vi "ShooterSim_Example.vi"() -> ()   [LabVIEW 2019]
uses:
  <vilib>/Rock Robotics/WPI/ThirdParty/JAS_Junk/TrajLib/DCMOTOR.CTL
  <vilib>/Rock Robotics/WPI/ThirdParty/JAS_Junk/TrajLib/LINEAR_SYSTEM.ctl
  <vilib>/Analysis/Matrix/Datatypes/RealMatrix.ctl
  <vilib>/Rock Robotics/WPI/ThirdParty/JAS_Junk/TrajLib/LINEAR_QUADRATIC_REGULATOR.ctl
  <vilib>/Rock Robotics/WPI/ThirdParty/JAS_Junk/TrajLib/KALMAN_FILTER.ctl
  <vilib>/Rock Robotics/WPI/ThirdParty/JAS_Junk/TrajLib/LINEAR_SYSTEM_LOOP.ctl
  <vilib>/Rock Robotics/WPI/ThirdParty/JAS_Junk/TrajLib/LINEAR_PLANT_INV_FF.ctl
  <vilib>/Rock Robotics/WPI/ThirdParty/JAS_Junk/TrajLib/FLYWHEEL_SIM.ctl
  <vilib>/Rock Robotics/WPI/ThirdParty/JAS_Junk/TrajLib/LINEAR_SYSTEM_SIM.ctl
  <vilib>/Rock Robotics/WPI/ThirdParty/JAS_Junk/TrajLib/DCMotor_New.vi
  <vilib>/Rock Robotics/WPI/ThirdParty/JAS_Junk/TrajLib/MatBuilder_Create.vi
  <vilib>/Rock Robotics/WPI/ThirdParty/JAS_Junk/TrajLib/LinearSystem_New.vi
  <vilib>/Rock Robotics/WPI/ThirdParty/JAS_Junk/TrajLib/MatrixHelper_Zero.vi
  <vilib>/Rock Robotics/WPI/ThirdParty/JAS_Junk/TrajLib/MatBuilder_Fill.vi
  <vilib>/Rock Robotics/WPI/ThirdParty/JAS_Junk/TrajLib/Matrix_Ident.vi
  <vilib>/Rock Robotics/WPI/ThirdParty/JAS_Junk/TrajLib/MatrixHelper_CoerceSize.vi
  <vilib>/Analysis/7linalg.llb/Create Special Matrix.vi
  <vilib>/Analysis/7linalg.llb/Create Special Real Matrix.vi
  <vilib>/Rock Robotics/WPI/ThirdParty/JAS_Junk/TrajLib/Trajectory_Library.lvlib
  <vilib>/Analysis/Matrix/NI_Matrix.lvlib
panel:
  in  "Tab Control":T1(tab)
  out "Motor Current":dbl format="%20.3f"
  out "Battery Voltage":dbl format="%20.3f"
  in  "Shoot ball":bool
  out "CO Chart":cluster{dbl, "Voltage":dbl}(graph)
  in  "Shooter On/Off":bool
  out "Encoer Speed\nRad/Sec":dbl(slide) scale=0.0..300.0
  out "Speed":dbl format="%20.3f"
  out "Cor Err":bool
  out "Kalman Filtered\nSpeed":dbl format="%20.3f"
  out "PV Chart":T2(graph)
  out "Predict Err":bool
  out "Motor Volt Dmd (CO)":dbl format="%20.3f"
  out "shoot Start":bool
  out "Shoot Done":bool
  out "Shooter Motor":T3 {"Jr_KgM2" format="%13.5p"; "L_H" format="%13.5p"; "Kt_NMPerAmp" format="%13.5p"; "KvINV_RadPerSecPerVolt" format="%13.5p"; "R_Ohms" format="%13.5p"; "FreeSpeed_RadPerSec" format="%13.5p"; "FreeCurrent_Amps" format="%13.5p"; "StallCurrent_Amps" format="%13.5p"; "StallTorque_NM" format="%13.5p"; "nominalVoltage_Volts" format="%13.5p"}
  out "m_flywheelPlant_ALT":T4
  out "m_FlyWheelSim":T6 {"GearBox"."Jr_KgM2" format="%13.5p"; "GearBox"."L_H" format="%13.5p"; "GearBox"."Kt_NMPerAmp" format="%13.5p"; "GearBox"."KvINV_RadPerSecPerVolt" format="%13.5p"; "GearBox"."R_Ohms" format="%13.5p"; "GearBox"."FreeSpeed_RadPerSec" format="%13.5p"; "GearBox"."FreeCurrent_Amps" format="%13.5p"; "GearBox"."StallCurrent_Amps" format="%13.5p"; "GearBox"."StallTorque_NM" format="%13.5p"; "GearBox"."nominalVoltage_Volts" format="%13.5p"}
  out "Shooting A":T5
  out "Shooting B":T5
  out "KalmanFilter":T8
  out "Kalman Error":errorcluster
  out "LinearQuadraticRegulator":T9
  out "LQR Error":bool
  out "Linear System Loop":T10
  out "LinSysLoop_Error":bool
  # "<States,States>"
  # "<States,Inputs>"
  # "<Outputs,States>"
  # "<Outputs,Inputs>"
  # "<States, 1>"
  # "<Outputs, 1>"
  # "<Inputs, 1>"
  # "<Outputs, 1>"
  # "<States,States>"
  # "<States,Inputs>"
  # "<Outputs,States>"
  # "<Outputs,Inputs>"
  # "Steady State Gain  \n<States,Outputs>"
  # "State Estimate <Statess,1>"
  # "<States,States>"
  # "<States,Inputs>"
  # "<Outputs,States>"
  # "<Outputs,Inputs>"
  # "Ref State <States,1>"
  # "Comp and capped \noutput <Inputs,1>"
  # "Controller gain\n<Inputs,States>"
  # "<States,1>"
  # "<FUTURE --- CLAMP TYPE -- For now\nuse Normalize>"
  # "Steady State Gain  \n<States,Outputs>"
  # "State Estimate <Statess,1>"
  # "<States,States>"
  # "<States,Inputs>"
  # "<Outputs,States>"
  # "<Outputs,Inputs>"
  # "<States,1>"
  # "<Inputs,1>"
  # "<States,Inputs>"
  # "<States,States>"
  # "Ref State <States,1>"
  # "Comp and capped \noutput <Inputs,1>"
  # "Controller gain\n<Inputs,States>"
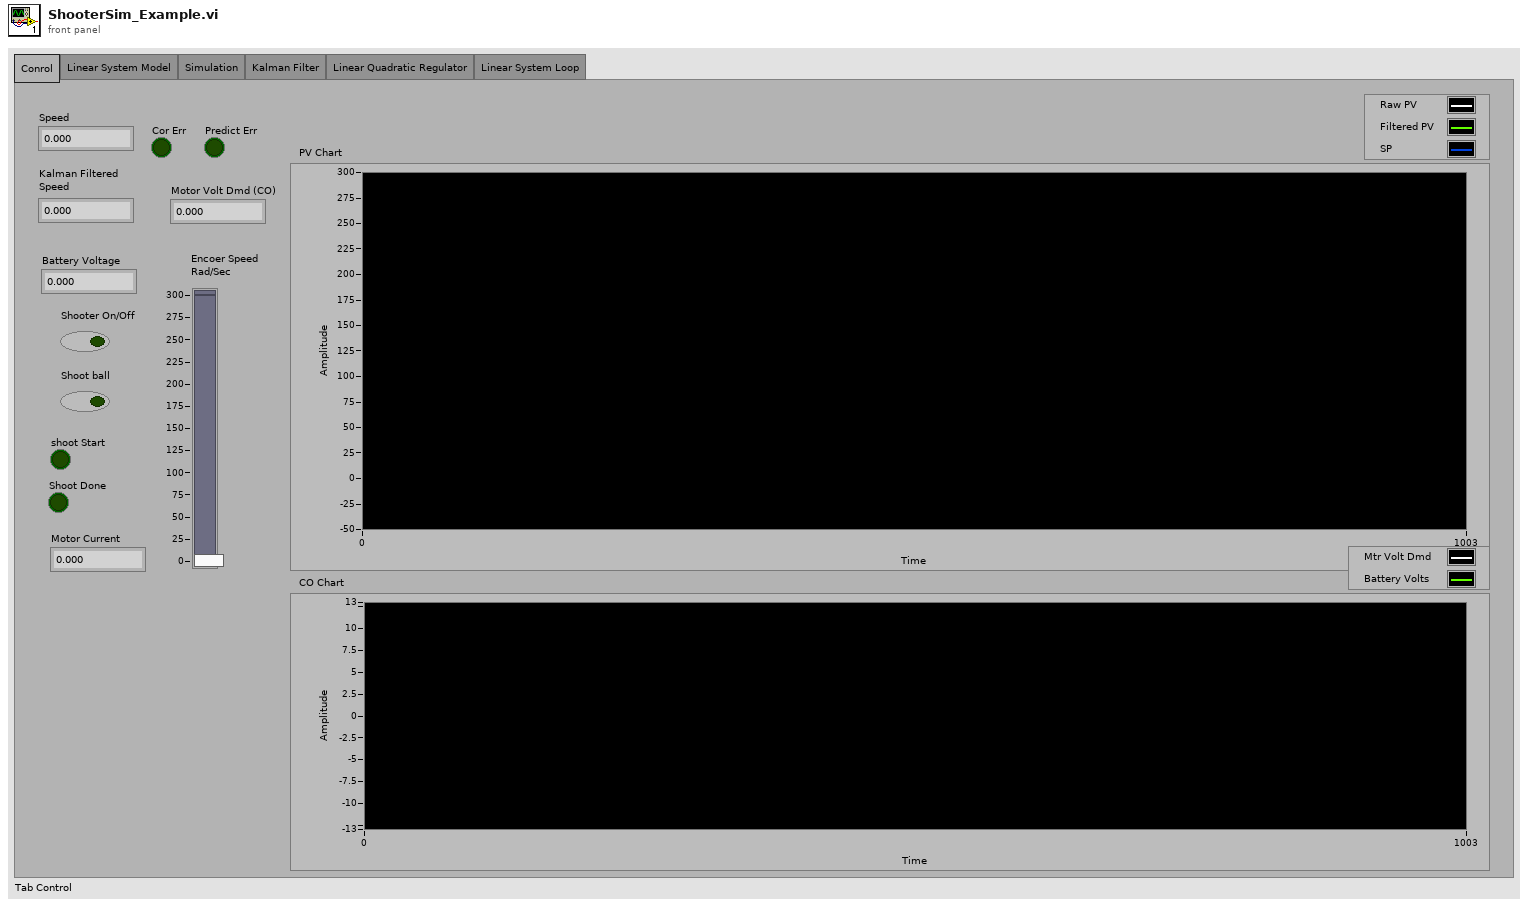
[diagram p1: front panel]
types:
  T1 = enum32{"Conrol", "Linear System Model", "Simulation", "Kalman Filter", "Linear Quadratic Regulator", "Linear System Loop"}
  T2 = cluster{"upper limit":dbl, "Real Matrix Element":dbl, "Real Matrix Element":dbl}
  T3 = typedef "Trajectory_Library.lvlib/DCMOTOR.CTL" = cluster{"nominalVoltage_Volts":dbl, "StallTorque_NM":dbl, "StallCurrent_Amps":dbl, "FreeCurrent_Amps":dbl, "FreeSpeed_RadPerSec":dbl, "R_Ohms":dbl, "KvINV_RadPerSecPerVolt":dbl, "Kt_NMPerAmp":dbl, "L_H":dbl, "Jr_KgM2":dbl}
  T4 = typedef "Trajectory_Library.lvlib/LINEAR_SYSTEM.ctl" = cluster{"m_A":T5, "m_B":T5, "m_C":T5, "m_D":T5, "States":i32, "Inputs":i32, "Outputs":i32}
  T5 = typedef "NI_Matrix.lvlib/RealMatrix.ctl" = dbl[][]
  T6 = typedef "Trajectory_Library.lvlib/FLYWHEEL_SIM.ctl" = cluster{"LinearSystemSim":T7, "GearBox":T3, "Gearing":dbl}
  T7 = typedef "Trajectory_Library.lvlib/LINEAR_SYSTEM_SIM.ctl" = cluster{"m_Plant":T4, "m_X":T5, "m_Y":T5, "m_U":T5, "MeasureStdDev":T5}
  T8 = typedef "Trajectory_Library.lvlib/KALMAN_FILTER.ctl" = cluster{"m_K":T5, "m_xHat":T5, "States":i32, "Outputs":i32, "m_Plant":T4}
  T9 = typedef "Trajectory_Library.lvlib/LINEAR_QUADRATIC_REGULATOR.ctl" = cluster{"m_r":T5, "m_U":T5, "m_K":T5, "States":i32, "Inputs":i32}
  T10 = typedef "Trajectory_Library.lvlib/LINEAR_SYSTEM_LOOP.ctl" = cluster{"Controller":T9, "FeedForward":T11, "Observer":T8, "Next_R":T5, "Clamp Max":T5}
  T11 = typedef "Trajectory_Library.lvlib/LINEAR_PLANT_INV_FF.ctl" = cluster{"m_R":T5, "m_Uff":T5, "m_B":T5, "m_A":T5, "States":i32, "Inputs":i32}
  T12 = cluster{"Velocity_RadPerSec":dbl, "Real Matrix Element":dbl, "Real Matrix Element":dbl}
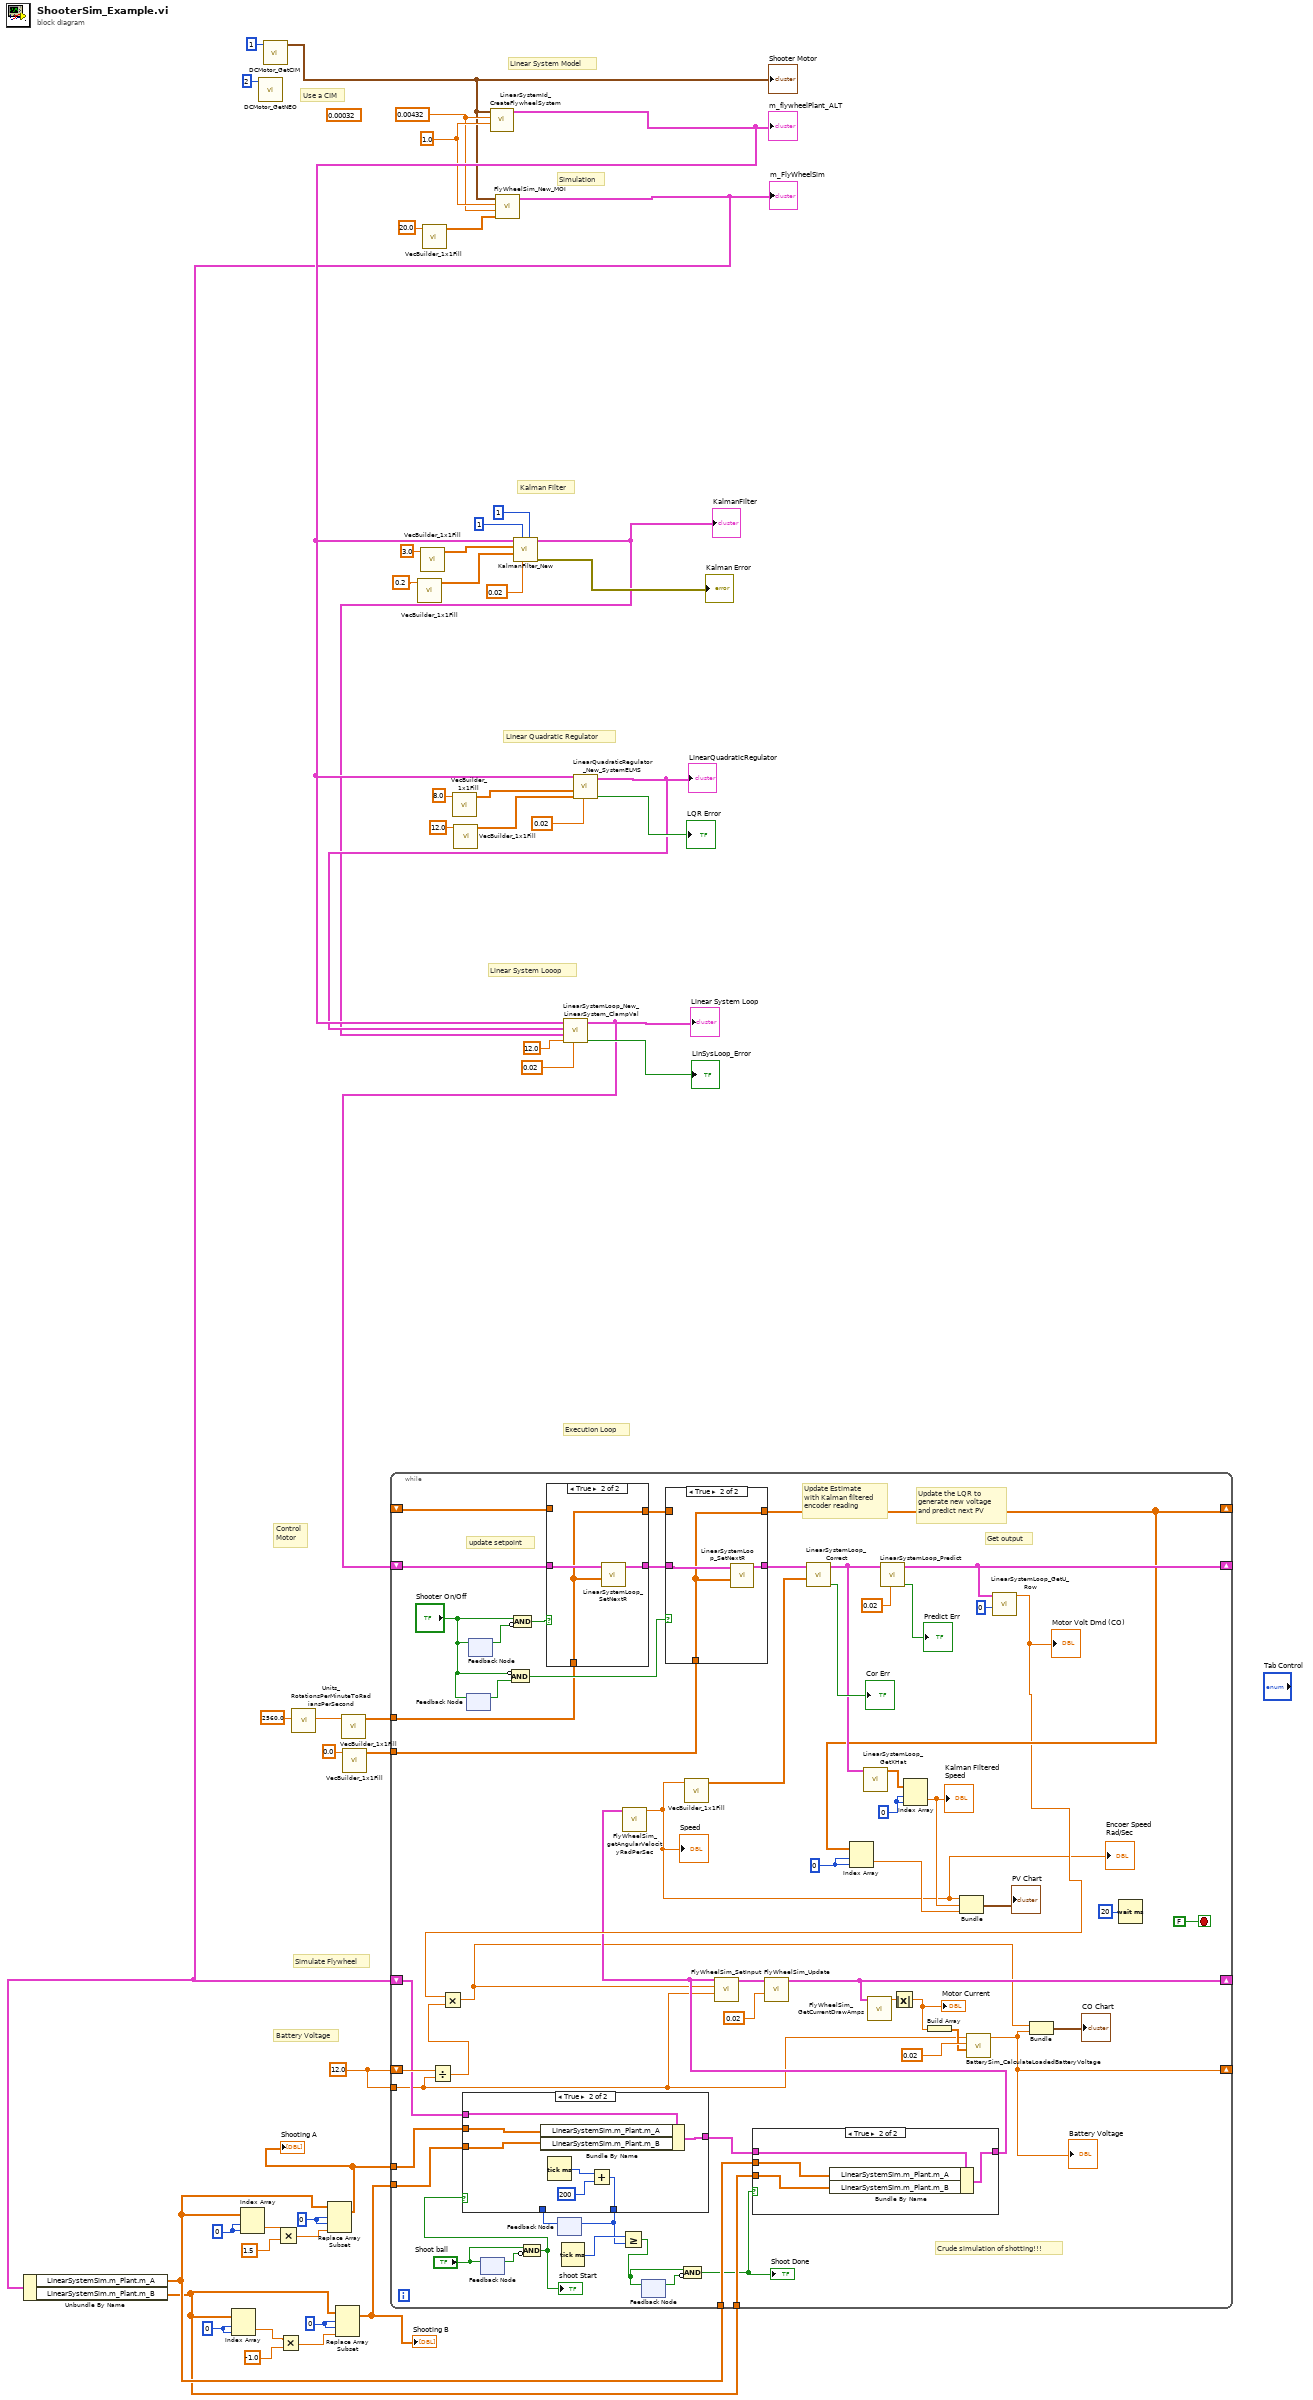
[diagram p0: block diagram]
diagram:
  w11 = 0 ("index (row)")
  w12 = 0 ("index (row)")
  w13 = 0 ("index (row)")
  w14 = 0 ("index (row)")
  w18 = 12.0
  w19 = 0.00432 ("jKgMetersSquared")
  w22 = 1.0 ("G")
  (unwired) 0.00032 ("jKgMetersSquared")
  # "Execution Loop"
  # "Linear System Looop"
  # "Linear Quadratic Regulator"
  # "Kalman Filter"
  # "Simulation"
  # "Linear System Model"
  # "Control\nMotor"
  # "Simulate Flywheel"
  # "Use a CIM"
  # "Battery Voltage"
  n1 = call <vilib>:"DCMotor_GetNEO.vi"("Num Motors"=2) -> ()  [unwired: 10 in, 1 out]
  n2 = call <vilib>:"DCMotor_GetCIM.vi"("Num Motors"=1) -> ("DCMOTOR"=w17:T3)  [unwired: 10 in]
  "Shooter Motor" <- w17
  n3 = call <vilib>:"Units_RotationsPerMinuteToRadiansPerSecond.vi"("RotationsPerMinute"=2560.0) -> ("RadiansPerSecond"=w26:dbl)  [unwired: 10 in]
  n4 = call <vilib>:"VecBuilder_1x1Fill.vi"("R0_C0"=w26) -> ("output matrix"=w24:T5)  [unwired: 10 in]
  n5 = call <vilib>:"VecBuilder_1x1Fill.vi"("R0_C0"=0.0) -> ("output matrix"=w23:T5)  [unwired: 10 in]
  n6 = call <vilib>:"VecBuilder_1x1Fill.vi"("R0_C0"=0.2) -> ("output matrix"=w36:T5)  [unwired: 10 in]
  n7 = call <vilib>:"VecBuilder_1x1Fill.vi"("R0_C0"=3.0) -> ("output matrix"=w37:T5)  [unwired: 10 in]
  n8 = call <vilib>:"VecBuilder_1x1Fill.vi"("R0_C0"=20.0) -> ("output matrix"=w21:T5)  [unwired: 10 in]
  n9 = call <vilib>:"VecBuilder_1x1Fill.vi"("R0_C0"=8.0) -> ("output matrix"=w45:T5)  [unwired: 10 in]
  n10 = call <vilib>:"VecBuilder_1x1Fill.vi"("R0_C0"=12.0) -> ("output matrix"=w43:T5)  [unwired: 10 in]
  n11 = call <vilib>:"LinearSystemId_CreateFlywheelSystem.vi"("G"=w22, "jKgMetersSquared"=w19, "DCMOTOR"=w17) -> ("Linearsystem"=w34:T4)  [unwired: 7 in, 1 out]
  "m_flywheelPlant_ALT" <- w34
  n12 = call <vilib>:"FlyWheelSim_New_MOI.vi"("MeasurementStdDev"=w21, "jKgMetersSquared"=w19, "Gearing"=w22, "GearBox"=w17) -> ("FlyWheelSim"=w15:T6)  [unwired: 6 in, 1 out]
  "m_FlyWheelSim" <- w15
  n13 = Unbundle By Name(w15) -> ("LinearSystemSim.m_Plant.m_A"=w4:T5, "LinearSystemSim.m_Plant.m_B"=w3:T5)
  n14 = Index Array(array=w3, index (row)=w14, index (col)=w14) -> (element=w6:dbl)
  n15 = Index Array(array=w4, index (row)=w13, index (col)=w13) -> (element=w10:dbl)
  n16 = Multiply(x=w10, y=1.5) -> (x*y=w8:dbl)
  n17 = Multiply(x=w6, y=-1.0) -> (x*y=w5:dbl)
  n18 = Replace Array Subset(array=w4, new element=w8, index (row)=w11, index (col)=w11) -> (w2:T5)
  "Shooting A" <- w2
  n19 = Replace Array Subset(array=w3, new element=w5, index (row)=w12, index (col)=w12) -> (w1:T5)
  "Shooting B" <- w1
  n20 = call <vilib>:"KalmanFilter_New.vi"("States"=1, "dt_Seconds"=0.02, "Outputs"=1, "MeasurementStdDevs"=w36, "StateStdDevs"=w37, "Plant"=w34) -> ("Error"=→"Kalman Error":errorcluster, "KalmanFilter"=w32:T8)  [unwired: 4 in]
  "KalmanFilter" <- w32
  n21 = call <vilib>:"LinearQuadraticRegulator_New_SystemELMS.vi"("dt_Seconds"=0.02, "Relms"=w43, "Qelms"=w45, "LINEARSYSTEM"=w34) -> ("Error"=→"LQR Error":bool, "LinearQuadraticRegulator"=w33:T9)  [unwired: 6 in]
  "LinearQuadraticRegulator" <- w33
  n22 = call <vilib>:"LinearSystemLoop_New_LinearSystem_ClampVal.vi"("dT_Seconds"=0.02, "Max_Voltage"=12.0, "Observer"=w32, "Controller"=w33, "Plant"=w34) -> ("Error"=→"LinSysLoop_Error":bool, "Linear System Loop"=w28:T10)  [unwired: 5 in]
  "Linear System Loop" <- w28
  n23 = while {
    shift-right: [w87] -> _
    shift-left: w28 -> [w101]
    tunnel: w24 -> [w99]
    tunnel: w23 -> [w98]
    shift-right: [w75] -> _
    shift-left: w15 -> [w70]
    shift-right: [w81] -> _
    shift-left: _ -> [w82]
    shift-right: [w71] -> _
    shift-left: w18 -> [w78]
    tunnel: w18 -> [w50]
    tunnel: w4 -> [w65]
    tunnel: w3 -> [w64]
    tunnel: w2 -> [w63]
    tunnel: w1 -> [w62]
    stop <- FALSE stop-if-true
    w80 = 0 ("index (row)")
    w94 = 0 ("index (row)")
    # "Crude simulation of shotting!!!"
    # "Get output"
    # "Update the LQR to \ngenerate new voltage\nand predict next PV"
    # "update setpoint"
    # "Update Estimate\nwith Kalman filtered\nencoder reading"
    n24 = Divide(x=w78, y=w50) -> (x/y=w76:dbl)
    n25 = feedback #1() -> (w105:bool)  [unwired: 1 in]
    n26 = feedback-in #1("Shooter On/Off") -> ()
    n27 = feedback-in #2("Shooter On/Off") -> ()
    n28 = feedback #2() -> (w106:bool)  [unwired: 1 in]
    n29 = feedback-in #3("Shoot ball") -> ()
    n30 = feedback #3() -> (w67:bool)  [unwired: 1 in]
    n31 = Compound Arithmetic op=AND(invert "Shooter On/Off", w105) -> (w102:bool)
    n32 = Compound Arithmetic op=AND("Shooter On/Off", invert w106) -> (w103:bool)
    n33 = Compound Arithmetic op=AND("Shoot ball", invert w67) -> (w66:bool)
    "shoot Start" <- w66
    n34 = case shown="True" w103 {
      tunnel: w101 -> [w129 w131]
      tunnel: [w129 w132] -> w100
      tunnel: w99 -> [_ w130]
      tunnel: [w128 w130] -> w83
      tunnel: w82 -> [w128 _]
      frame False {
      }
      frame True {
        n35 = call <vilib>:"LinearSystemLoop_SetNextR.vi"("R"=w130, "input inear System Loop"=w131) -> ("out Linear System Loop"=w132:T10)  [unwired: 8 in, 1 out]
      }
    }
    n36 = feedback #4() -> (w56:u32)  [unwired: 1 in]
    n37 = case shown="True" w66 {
      tunnel: w70 -> [w115 w122]
      tunnel: [w115 w119] -> w69
      tunnel: w63 -> [_ w121]
      tunnel: w62 -> [_ w120]
      tunnel: [w114 w116] -> w57
      tunnel: w56 -> [w114 _]
      frame False {
      }
      frame True {
        n38 = Bundle By Name(cluster=w122, "LinearSystemSim.m_Plant.m_A"=w121, "LinearSystemSim.m_Plant.m_B"=w120) -> (w119:T6)
        n39 = Tick Count (ms)() -> (millisecond timer value=w118:u32)
        n40 = Add(x=w118, y=u32 200) -> (x+y=w116:u32)
      }
    }
    n41 = feedback-in #4(w57) -> ()
    n42 = Tick Count (ms)() -> (millisecond timer value=w61:u32)
    n43 = Greater Or Equal?(x=w61, y=w57) -> (x >= y?=w59:bool)
    n44 = feedback #5() -> (w60:bool)  [unwired: 1 in]
    n45 = feedback-in #5(w59) -> ()
    n46 = case shown="True" w102 {
      tunnel: w100 -> [w124 w126]
      tunnel: [w124 w127] -> w97
      tunnel: w98 -> [_ w125]
      tunnel: w83 -> [w123 _]
      tunnel: [w123 w125] -> w81
      frame False {
      }
      frame True {
        n47 = call <vilib>:"LinearSystemLoop_SetNextR.vi"("R"=w125, "input inear System Loop"=w126) -> ("out Linear System Loop"=w127:T10)  [unwired: 8 in, 1 out]
      }
    }
    n48 = Compound Arithmetic op=AND(w59, invert w60) -> (w58:bool)
    "Shoot Done" <- w58
    n49 = case shown="True" w58 {
      tunnel: w69 -> [w109 w113]
      tunnel: [w109 w112] -> w53
      tunnel: w65 -> [_ w111]
      tunnel: w64 -> [_ w110]
      frame False {
      }
      frame True {
        n50 = Bundle By Name(cluster=w113, "LinearSystemSim.m_Plant.m_A"=w111, "LinearSystemSim.m_Plant.m_B"=w110) -> (w112:T6)
      }
    }
    n51 = call <vilib>:"FlyWheelSim_getAngularVelocityRadPerSec.vi"("FlyWheelSim"=w53) -> ("Velocity_RadPerSec"=w52:dbl)  [unwired: 10 in]
    "Encoer Speed\nRad/Sec" <- w52
    "Speed" <- w52
    n52 = call <vilib>:"VecBuilder_1x1Fill.vi"("R0_C0"=w52) -> ("output matrix"=w96:T5)  [unwired: 10 in]
    n53 = call <vilib>:"LinearSystemLoop_Correct.vi"("Y"=w96, "input inear System Loop"=w97) -> ("Error"=→"Cor Err":bool, "out Linear System Loop"=w90:T10)  [unwired: 8 in]
    n54 = Index Array(array=w81, index (row)=w80, index (col)=w80) -> (element=w79:dbl)
    n55 = call <vilib>:"LinearSystemLoop_GetXHat.vi"("input inear System Loop"=w90) -> ("XHat"=w93:T5)  [unwired: 10 in]
    n56 = call <vilib>:"LinearSystemLoop_Predict.vi"("dT_Seconds"=0.02, "input inear System Loop"=w90) -> ("Error"=→"Predict Err":bool, "out Linear System Loop"=w87:T10)  [unwired: 8 in]
    n57 = Index Array(array=w93, index (row)=w94, index (col)=w94) -> (element=w92:dbl)
    "Kalman Filtered\nSpeed" <- w92
    n58 = Bundle("Velocity_RadPerSec"=w52, "Real Matrix Element"=w92, "Real Matrix Element"=w79) -> (→"PV Chart":T12)  [unwired: 1 in]
    n59 = call <vilib>:"LinearSystemLoop_GetU_Row.vi"("Row"=0, "input inear System Loop"=w87) -> ("U"=w77:dbl)  [unwired: 9 in]
    "Motor Volt Dmd (CO)" <- w77
    n60 = Multiply(x=w77, y=w76) -> (x*y=w51:dbl)
    n61 = call <vilib>:"FlyWheelSim_SetInput.vi"("Battery_Volts"=w50, "Volts"=w51, "FlyWheelSim"=w53) -> ("out FlyWheelSim"=w85:T6)  [unwired: 8 in]
    n62 = call <vilib>:"FlyWheelSim_Update.vi"("dT_Seconds"=0.02, "FlyWheelSim"=w85) -> ("out FlyWheelSim"=w75:T6)  [unwired: 8 in, 1 out]
    n63 = call <vilib>:"FlyWheelSim_GetCurrentDrawAmps.vi"("FlyWheelSim"=w75) -> ("Current_Amps"=w55:dbl)  [unwired: 10 in]
    n64 = Absolute Value(x=w55) -> (abs(x)=w54:dbl)
    "Motor Current" <- w54
    n65 = Build Array(w54) -> (w73:dbl[])
    n66 = call <vilib>:"BatterySim_CalculateLoadedBatteryVoltage.vi"("Currents"=w73, "Resistance_Ohms"=0.02, "NominalVoltage"=w50) -> ("Voltage"=w71:dbl)  [unwired: 8 in]
    "Battery Voltage" <- w71
    n67 = Bundle(w51, "Voltage"=w71) -> (→"CO Chart":cluster{dbl, "Voltage":dbl})  [unwired: 1 in]
    n68 = Wait (ms)(milliseconds to wait=u32 20) -> ()  [unwired: 1 out]
  }
